vi "Output Panel Init.vi"(8 "error in (no error)":errorcluster, 10 "Size":i32, 11 "VI in":refnum<vi>) -> (0 "error out":errorcluster, 3 "Entry Panel out":refnum<vi>[](array[refnum]))   [LabVIEW 2015, in "OutputUI.lvclass"]
uses:
  OutputUI.lvclass
  <vilib>/Utility/miscctls.llb/LVPointTypeDef.ctl
  <vilib>/Utility/miscctls.llb/LVPositionTypeDef.ctl
  <vilib>/Utility/miscctls.llb/LVBoundsTypeDef.ctl
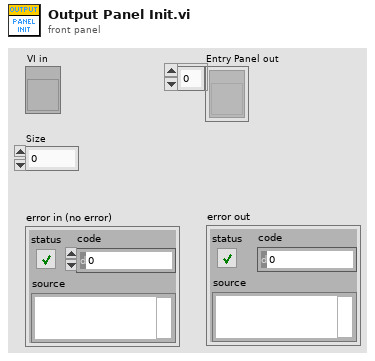
[diagram p1: front panel]
types:
  T1 = typedef "LVPointTypeDef.ctl" = cluster{"Horizontal":i16, "Vertical":i16}
  T2 = typedef "LVPositionTypeDef.ctl" = cluster{"Left":i32, "Top":i32}
  T3 = typedef "LVBoundsTypeDef.ctl" = cluster{"Width":u32, "Height":u32}
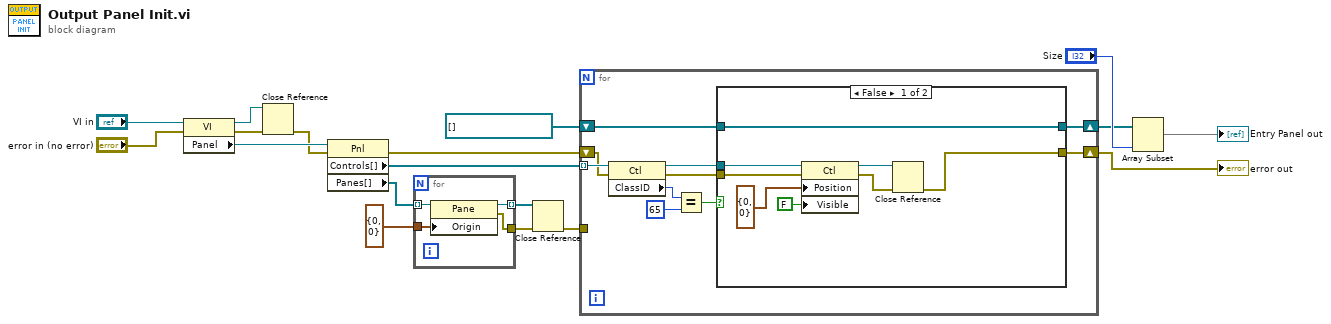
[diagram p0: block diagram]
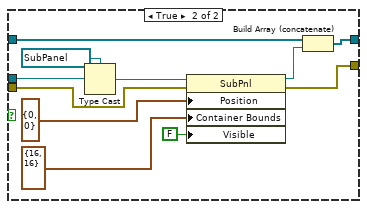
[diagram p2: hidden frame]
diagram:
  n1 = property class="VI"(reference="VI in", error in="error in (no error)") -> (reference out=w2:refnum<vi>, error out=w3:errorcluster, "Panel"=w9:refnum<vi>)
  n2 = Close Reference(reference=w2, error in (no error)=w3) -> (error out=w1:errorcluster)
  n3 = property class="Pnl"(reference=w9, error in=w1) -> (error out=w7:errorcluster, "Controls[]"=w8:refnum<vi>[], "Panes[]"=w11:refnum<vi>[])  [unwired: 1 out]
  n4 = for {
    tunnel: w11 -> [w22] mode=indexing
    tunnel: T1 {"Horizontal"=0, "Vertical"=0} ("Origin") -> [w21]
    tunnel: [w20] -> w13 mode=indexing
    tunnel: [w19] -> w14
    n5 = property class="Pane"(reference=w22, "Origin"=w21) -> (reference out=w20:refnum<vi>, error out=w19:errorcluster)  [unwired: 1 in]
  }
  n6 = Close Reference(reference=w13, error in (no error)=w14) -> (error out=w15:errorcluster)
  n7 = for {
    tunnel: w8 -> [w32] mode=indexing
    shift-right: [w25] -> w5
    shift-left: w7 -> [w27]
    shift-right: [w24] -> w16
    shift-left: refnum<vi>[] [] -> [w23]
    tunnel: w15 -> [_]
    n8 = property class="Ctl"(reference=w32, error in=w27) -> (reference out=w31:refnum<vi>, error out=w26:errorcluster, "ClassID"=w29:u32)
    n9 = Equal?(x=w29, y=65) -> (x = y?=w28:bool)
    n10 = case shown="False" w28 {
      tunnel: w31 -> [w39 w49]
      tunnel: w26 -> [w38 w46]
      tunnel: [w35 w44] -> w25
      tunnel: [w40 w42] -> w24
      tunnel: w23 -> [w40 w41]
      frame False {
        n11 = property class="Ctl"(reference=w39, error in=w38, "Position"=T2 {"Left"=0, "Top"=0}, "Visible"=FALSE) -> (reference out=w37:refnum<vi>, error out=w36:errorcluster)
        n12 = Close Reference(reference=w37, error in (no error)=w36) -> (error out=w35:errorcluster)
      }
      frame True {
        n13 = Type Cast(type=refnum<vi> refnum ("reference out"), x=w49) -> (*(type *) &x=w48:refnum<vi>)
        n14 = property class="SubPnl"(reference=w48, error in=w46, "Position"=T2 {"Left"=0, "Top"=0}, "Container Bounds"=T3 {"Width"=16, "Height"=16} ("XControl:Container Bounds"), "Visible"=FALSE) -> (reference out=w43:refnum<vi>, error out=w44:errorcluster)
        n15 = Build Array (concatenate)(w41, w43) -> (w42:refnum<vi>[])
      }
    }
  }
  "error out" <- w5
  n16 = Array Subset(array=w16, length="Size") -> (→"Entry Panel out":refnum<vi>[])  [unwired: 1 in]
